vi "Configure Multi Eval Meas Limit IQ Offset.vi"(0 "VISA resource name":refnum<visa-resource-name>, 1 "Offset 0 (-2.6)":dbl=-2.6 format="%^.3e", 2 "Offset 2 (0.0)":dbl format="%^.3e", 5 "Instance (1)":T1=1, 7 "Modulation (Pi/2-BPSK)":i32(ring) items=["Pi/2-BPSK", "Pi/2-BPSK With Shaping", "QPSK", "16-QAM", "64-QAM", "256-QAM"], 9 "Enabled (Off)":bool, 11 "error in (no error)":errorcluster, 12 "Offset 1 (2.1)":dbl=2.1 format="%^.3e", 13 "Offset 3 (0.0)":dbl format="%^.3e") -> (4 "VISA resource name out":refnum<visa-resource-name>, 15 "error out":errorcluster)   [LabVIEW 2020, in "Rohde&Schwarz CMWXP NR FR1 Measurement.lvlib"]
doc: "Defines upper limits for the I/Q origin offset. Two different I/Q origin offset limits can be set for two TX power ranges.\n\nAttributes:\nRSCMWXPNRFR1M_ATTR_MULTI_EVAL_MEAS_LIMIT_PI_2_IQ_OFFSET\nRSCMWXPNRFR1M_ATTR_MULTI_EVAL_MEAS_LIMIT_BPSK_SHAPING_IQ_OFFSET\nRSCMWXPNRFR1M_ATTR_MULTI_EVAL_MEAS_LIMIT_QPSK_IQ_OFFSET\nRSCMWXPNRFR1M_ATTR_MULTI_EVAL_MEAS_LIMIT_QAM_IQ_OFFSET\n\nRemote-control commands:\nCONFigure:NRSub:MEAS<i>:MEValuation:LIMit:PHBPsk:IQOFfset\nCONFigure:NRSub:MEAS<i>:MEValuation:LIMit:BPWShaping:IQOFfset\nCONFigure:NRSub:MEAS<i>:MEValuation:LIMit:QPSK:IQOFfset\nCONFigure:NRSub:MEAS<i>:MEValuation:LIMit:QAM<order>:IQOFfset"
uses:
  <instrlib>/Rohde&Schwarz CMWXP NR FR1 Measurement/Rohde&Schwarz CMWXP NR FR1 Measurement.lvlib
  <instrlib>/Rohde&Schwarz CMWXP NR FR1 Measurement/Private/_Instance.ctl
  <instrlib>/Rohde&Schwarz CMWXP NR FR1 Measurement/Private/rsidr_core.llb/rsidr_core.lvlib
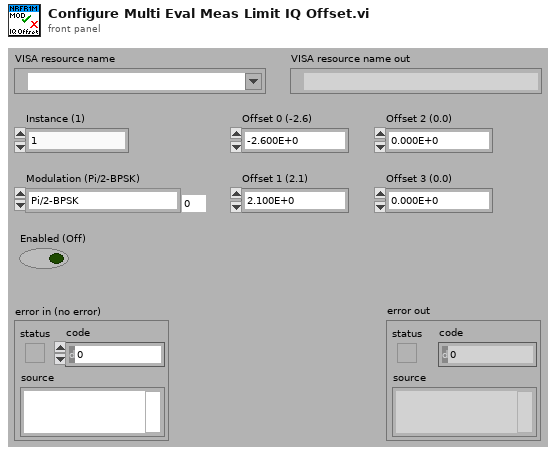
[diagram p1: front panel]
types:
  T1 = typedef "Rohde&Schwarz CMWXP NR FR1 Measurement.lvlib/_Instance.ctl" = i32
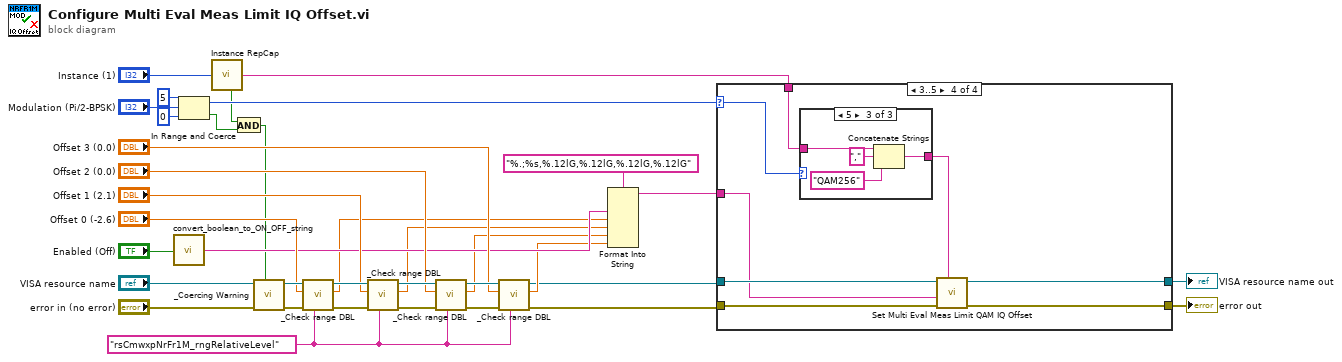
[diagram p0: block diagram]
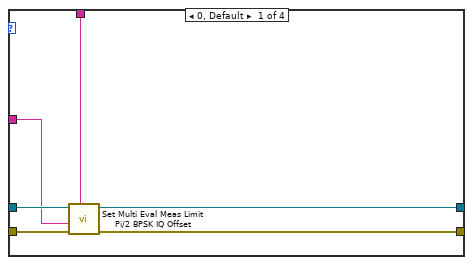
[diagram p2: hidden frame]
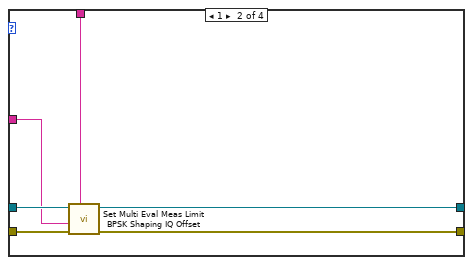
[diagram p3: hidden frame]
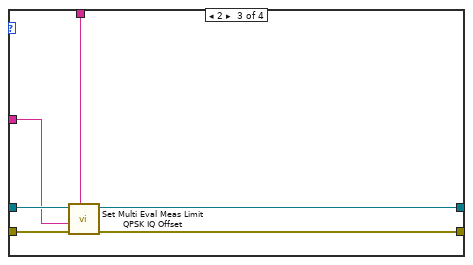
[diagram p4: hidden frame]
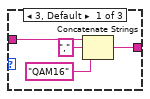
[diagram p5: hidden frame]
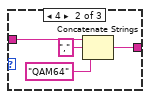
[diagram p6: hidden frame]
diagram:
  w17 = "rsCmwxpNrFr1M_rngRelativeLevel" ("Range Table Identifier")
  n1 = call <instrlib>:"convert_boolean_to_ON_OFF_string.vi"("boolean value in"="Enabled (Off)") -> ("string value out"=w15:string)  [unwired: 4 in]
  n2 = In Range and Coerce(upper limit=5, x="Modulation (Pi/2-BPSK)", lower limit=0) -> (coerced(x)=w7:i32, In Range?=w2:bool)
  n3 = call <instrlib>:"Instance RepCap.vi"("Instance In"="Instance (1)") -> ("In Range?"=w1:bool, "RepCap Identifier Out"=w6:string)  [unwired: 1 in]
  n4 = And(x=w1, y=w2) -> (x .and. y?=w3:bool)
  n5 = call <instrlib>:"_Coercing Warning.vi"("In Range?"=w3, "error in (no error)"="error in (no error)", "VISA resource name"="VISA resource name") -> ("error out"=w29:errorcluster, "VISA resource name out"=w28:refnum<visa-resource-name>)  [unwired: 7 in]
  n6 = call <instrlib>:"_Check range DBL.vi"("Range Table Identifier"=w17, "error in (no error)"=w29, "DBL Value In"="Offset 0 (-2.6)", "VISA resource name"=w28) -> ("error out"=w27:errorcluster, "DBL Value Out"=w14:dbl, "VISA resource name out"=w26:refnum<visa-resource-name>)  [unwired: 5 in]
  n7 = call <instrlib>:"_Check range DBL.vi"("Range Table Identifier"=w17, "error in (no error)"=w27, "DBL Value In"="Offset 1 (2.1)", "VISA resource name"=w26) -> ("error out"=w25:errorcluster, "DBL Value Out"=w13:dbl, "VISA resource name out"=w24:refnum<visa-resource-name>)  [unwired: 5 in]
  n8 = call <instrlib>:"_Check range DBL.vi"("Range Table Identifier"=w17, "error in (no error)"=w25, "DBL Value In"="Offset 2 (0.0)", "VISA resource name"=w24) -> ("error out"=w23:errorcluster, "DBL Value Out"=w12:dbl, "VISA resource name out"=w22:refnum<visa-resource-name>)  [unwired: 5 in]
  n9 = call <instrlib>:"_Check range DBL.vi"("Range Table Identifier"=w17, "error in (no error)"=w23, "DBL Value In"="Offset 3 (0.0)", "VISA resource name"=w22) -> ("error out"=w9:errorcluster, "DBL Value Out"=w11:dbl, "VISA resource name out"=w10:refnum<visa-resource-name>)  [unwired: 5 in]
  n10 = Format Into String(format string="%.;%s,%.12lG,%.12lG,%.12lG,%.12lG", w15, w14, w13, w12, w11) -> (resulting string=w8:string)  [unwired: 2 in, 1 out]
  n11 = case shown="3..5" w7 {
    selector: w7 -> [_ _ _ w57]
    tunnel: w9 -> [w42 w48 w54 w62]
    tunnel: [w41 w47 w53 w61] -> w4
    tunnel: [w40 w46 w52 w60] -> w5
    tunnel: w10 -> [w39 w45 w51 w59]
    tunnel: w6 -> [w38 w44 w50 w56]
    tunnel: w8 -> [w37 w43 w49 w58]
    frame 0, Default {
      n12 = call "Set Multi Eval Meas Limit Pi/2 BPSK IQ Offset"("Repeated Capabilities"=w38, "error in (no error)"=w42, "Multi Eval Meas Limit Pi/2 BPSK IQ Offset ()"=w37, "instrument handle"=w39) -> ("error out"=w41:errorcluster, "instrument handle out"=w40:refnum<visa-resource-name>)  [unwired: 6 in]
    }
    frame 1 {
      n13 = call "Set Multi Eval Meas Limit BPSK Shaping IQ Offset"("Repeated Capabilities"=w44, "error in (no error)"=w48, "Multi Eval Meas Limit BPSK Shaping IQ Offset ()"=w43, "instrument handle"=w45) -> ("error out"=w47:errorcluster, "instrument handle out"=w46:refnum<visa-resource-name>)  [unwired: 6 in]
    }
    frame 2 {
      n14 = call "Set Multi Eval Meas Limit QPSK IQ Offset"("Repeated Capabilities"=w50, "error in (no error)"=w54, "Multi Eval Meas Limit QPSK IQ Offset ()"=w49, "instrument handle"=w51) -> ("error out"=w53:errorcluster, "instrument handle out"=w52:refnum<visa-resource-name>)  [unwired: 6 in]
    }
    frame 3..5 {
      n15 = case shown="5" w57 {
        tunnel: w56 -> [w66 w70 w74]
        tunnel: [w65 w69 w73] -> w55
        frame 3, Default {
          n16 = Concatenate Strings(w66, "," ("string"), "QAM16" ("string")) -> (w65:string)
        }
        frame 4 {
          n17 = Concatenate Strings(w70, "," ("string"), "QAM64" ("string")) -> (w69:string)
        }
        frame 5 {
          n18 = Concatenate Strings(w74, "," ("string"), "QAM256" ("string")) -> (w73:string)
        }
      }
      n19 = call "Set Multi Eval Meas Limit QAM IQ Offset"("Repeated Capabilities"=w55, "error in (no error)"=w62, "Multi Eval Meas Limit QAM IQ Offset ()"=w58, "instrument handle"=w59) -> ("error out"=w61:errorcluster, "instrument handle out"=w60:refnum<visa-resource-name>)  [unwired: 6 in]
    }
  }
  "error out" <- w4
  "VISA resource name out" <- w5
